vi "Begin.vi"(8 "error in":errorcluster) -> (0 "error out":errorcluster)   [LabVIEW 2020]
doc: "Called before other user functions, this VI is expected to open initial I/O refnums, load in file data, and do all program initialization. Notice that the <B>error out</B> terminal is simply used for data flow. Wiring it to other structures or subVIs ensures that this VI runs first."
uses:
  <vilib>/Rock Robotics/WPI/DriverStation/WPI_DriverStationRobotMode2.ctl
  <vilib>/Rock Robotics/WPI/Joystick/WPI_JoystickDeviceEnum.ctl
  <vilib>/Rock Robotics/WPI/ThirdParty/REV Robotics/REVLib/Typedef/Spark MAX Sensor Type.ctl
  <vilib>/Rock Robotics/WPI/SafetyOutput/WPI_SafetyOutputConfigMenu.ctl
  <vilib>/Rock Robotics/WPI/ThirdParty/REV Robotics/REVLib/Typedef/Spark MAX Motor Type.ctl
  Robot Global Data.vi
  <vilib>/Rock Robotics/Network Tables/NT Write String Array.vi
  <vilib>/Rock Robotics/WPI/RobotDrive/WPI_RobotDriveOpen2MotorWithExistingMotors.vi
  <vilib>/Rock Robotics/SystemInterfaces/DIO/FPGA_DIOPWMChannel.ctl
  <vilib>/Rock Robotics/WPI/RobotDrive/WPI_RobotDriveOpen2MotorWithVictorSPX.vi
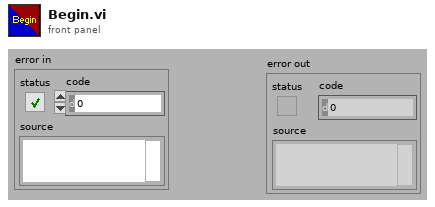
[diagram p1: front panel]
types:
  T1 = typedef "WPI_JoystickDeviceEnum.ctl" = enum16{"USB 0", "USB 1", "USB 2", "USB 3", "USB 4", "USB 5"}
  T2 = typedef "Spark MAX Motor Type.ctl" = enum16{"Brushed", "Brushless"}
  T3 = typedef "WPI_SafetyOutputConfigMenu.ctl" = enum16{"Enable", "Disable"}
  T4 = typedef "Spark MAX Sensor Type.ctl" = enum16{"No Sensor", "Hall Sensor", "Encoder", "-Not Available-", "Analog", "Alternate Encoder", "Duty Cycle"}
  T5 = typedef "WPI_DriverStationRobotMode2.ctl" = enum16{"Autonomous Disabled", "Autonomous Enabled", "Teleop Disabled", "Teleop Enabled", "Disconnected", "Finish", "Test Disabled", "Test Enabled", "Emergency Stopped"}
  T6 = typedef "FPGA_DIOPWMChannel.ctl" = enum8{"PWM 0", "PWM 1", "PWM 2", "PWM 3", "PWM 4", "PWM 5", "PWM 6", "PWM 7", "PWM 8", "PWM 9", "PWM MXP 0", "PWM MXP 1", "PWM MXP 2", "PWM MXP 3", "PWM MXP 4", "PWM MXP 5", "PWM MXP 6", "PWM MXP 7", "PWM MXP 8", "PWM MXP 9", "Invalid"}
  T7 = typedef "WPI_RobotDriveDevRef.ctl" = cluster{"DevStatus":errorcluster, "Motors[]":T8[], "Square Inputs":bool, "Max Output":dbl}
  T8 = typedef "WPI_MotorControlDeviceRef.ctl" = cluster{"DeviceStatus":errorcluster, "Type":T9, "PWM":cluster{"PWM Channel":T6, "DeadBand":T10}, "CAN":cluster{"Device Number":u8, "SetOutput VI Ref":variant, "GetOutput VI Ref":variant, "Enable VI Ref":variant, "Disable VI Ref":variant, "Data":variant}, "Invert":bool, "DIO PWM":cluster{"PWM \"Enable\" Channel":T6, "DIOChannel":T11, "PWM Rate":dbl}}
  T9 = typedef "WPI_MotorControlType.ctl" = enum16{"PWM", "CAN", "DIO PWM"}
  T10 = typedef "WPI_PWMDeadband.ctl" = cluster{"Name":string, "maxPositivePwm":i32, "minPositivePwm":i32, "centerPwm":i32, "maxNegativePwm":i32, "minNegativePwm":i32, "angularRange":u16}
  T11 = typedef "FPGA_DIOChannel.ctl" = enum8{"DIO 0", "DIO 1", "DIO 2", "DIO 3", "DIO 4", "DIO 5", "DIO 6", "DIO 7", "DIO 8", "DIO 9", "DIO MXP 0", "DIO MXP 1", "DIO MXP 2", "DIO MXP 3", "DIO MXP 4", "DIO MXP 5", "DIO MXP 6", "DIO MXP 7", "DIO MXP 8", "DIO MXP 9", "DIO MXP 10", "DIO MXP 11", "DIO MXP 12", "DIO MXP 13", "DIO MXP 14", "DIO MXP 15", "SPI Port CS1", "SPI Port CS2", "SPI Port CS3", "SPI Port MISO", "SPI Port MOSI", "Invalid"}
  T12 = typedef "WPI_JoystickDevRef.ctl" = cluster{"Device":T1}
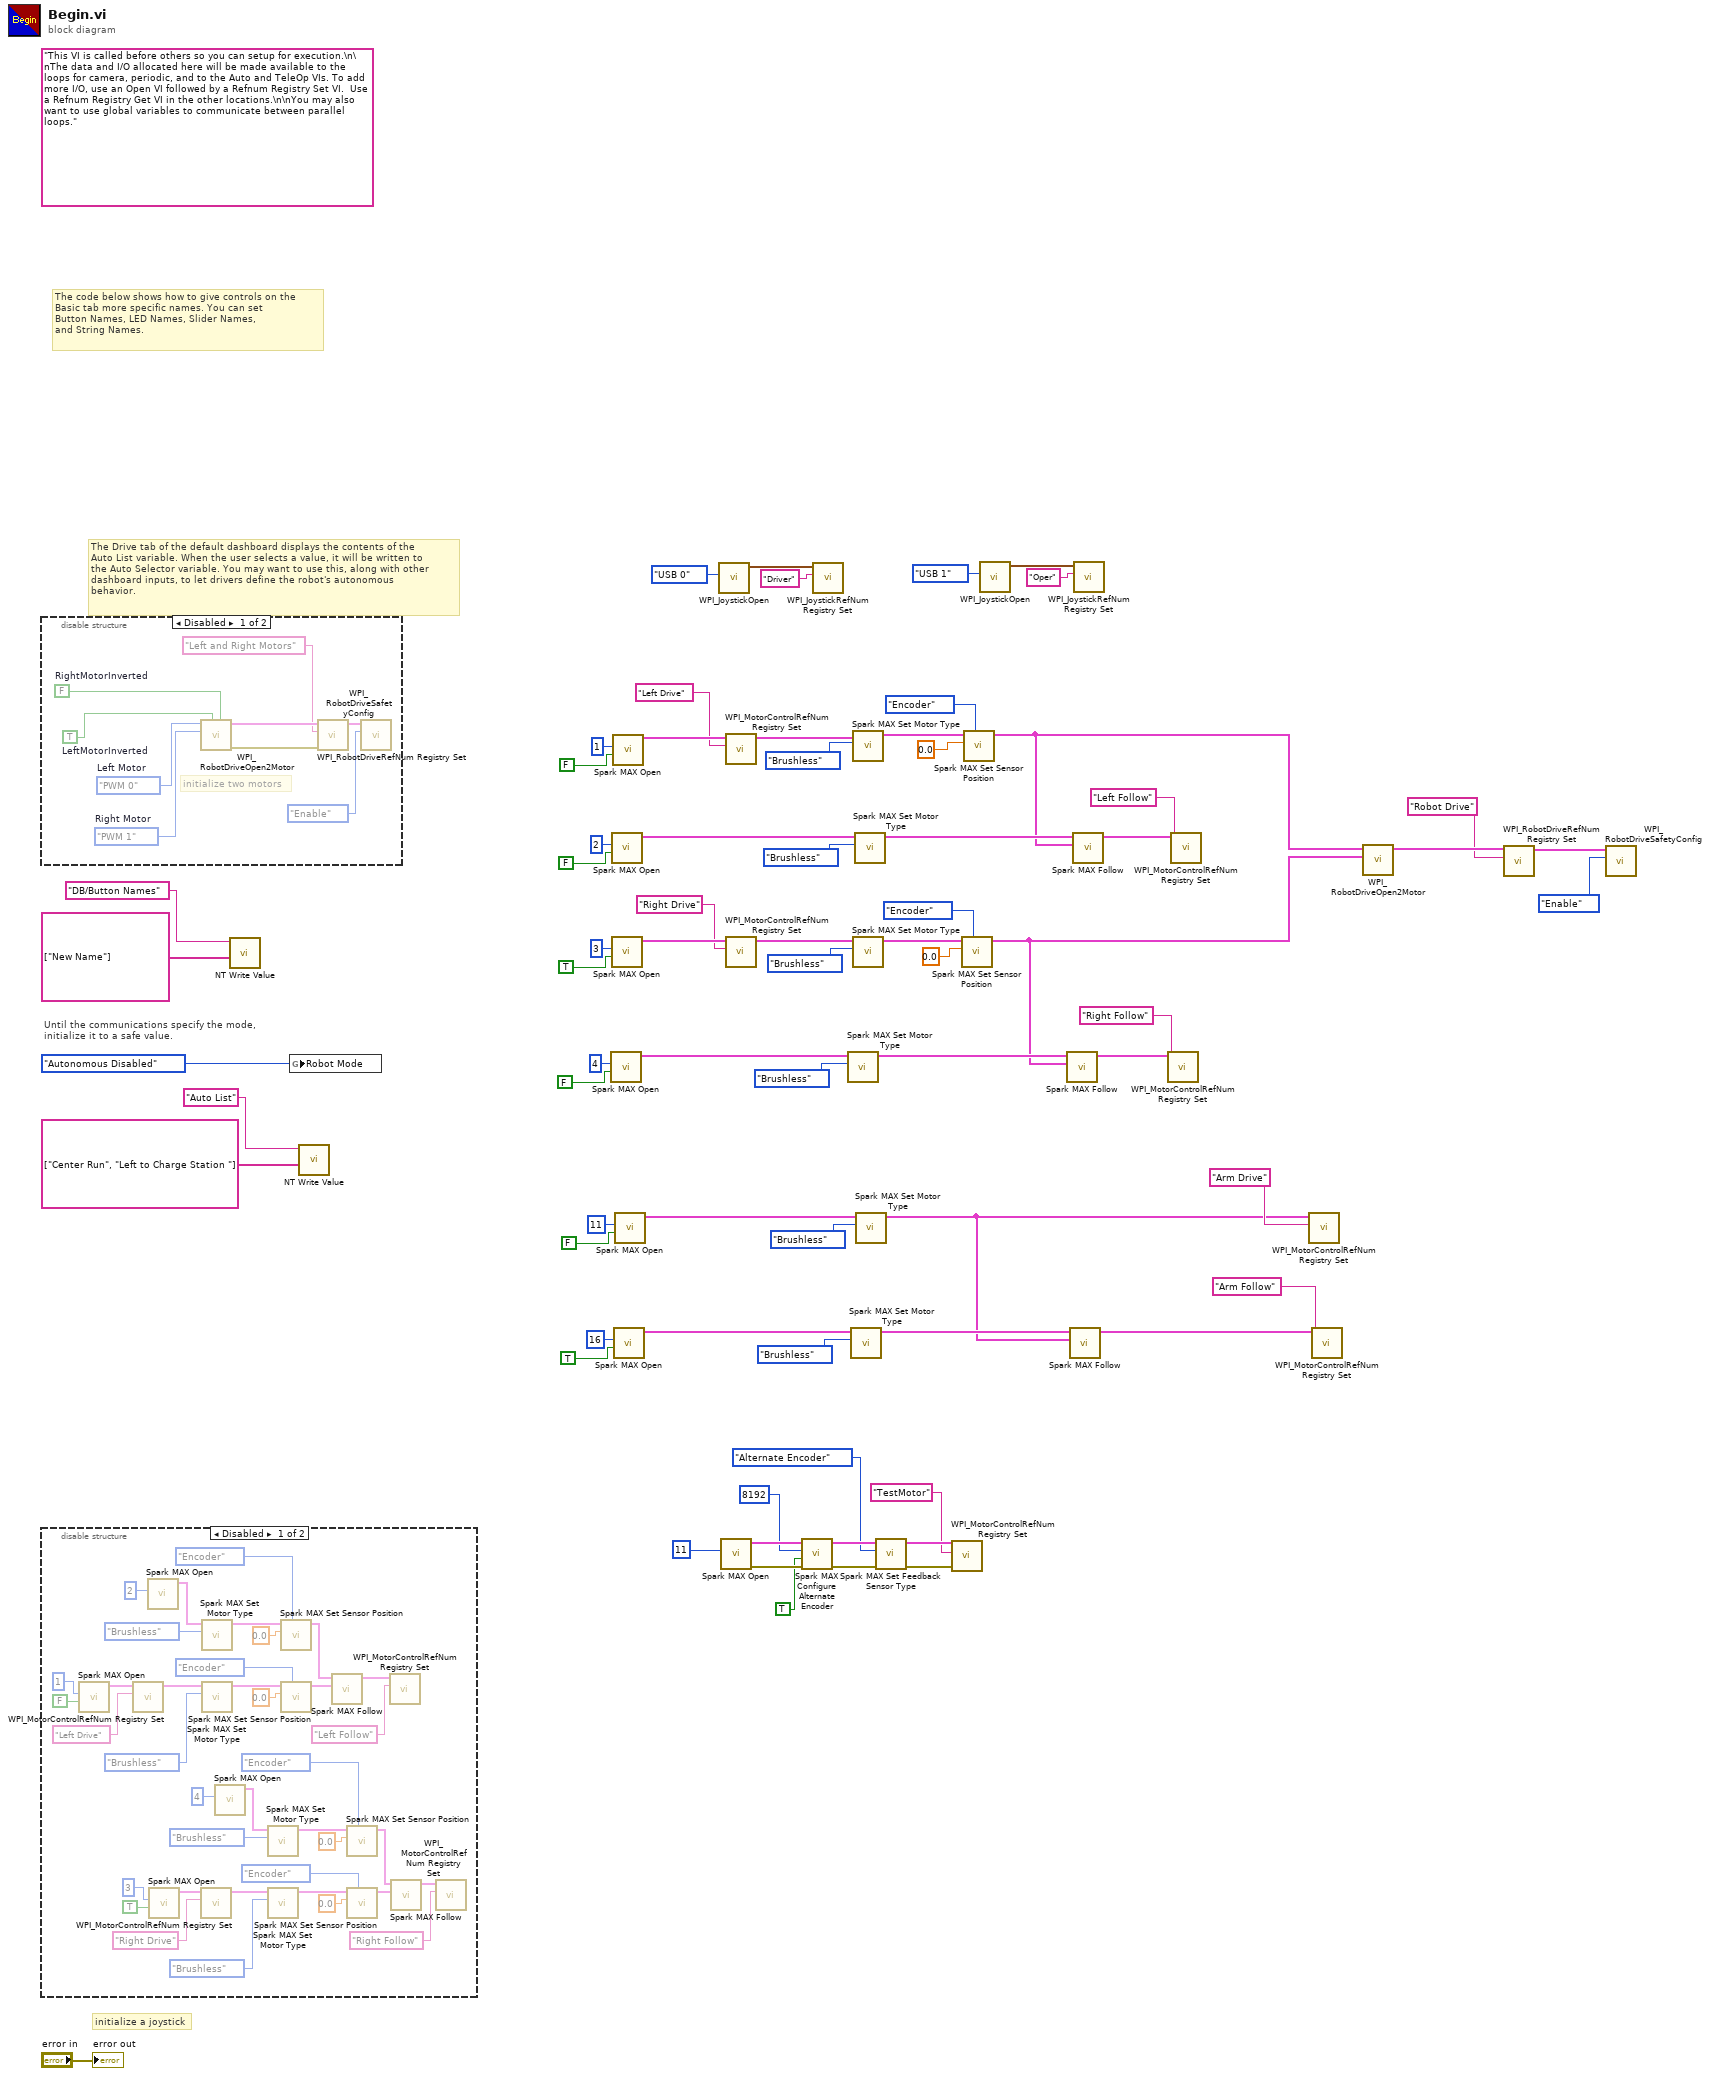
[diagram p0: block diagram]
diagram:
  (unwired) "This VI is called before others so you can setup for execution.\n\nThe data and I/O allocated here will be made available to the loops for camera, periodic, and to the Auto and TeleOp VIs. To add more I/O, use an Open VI followed by a Refnum Registry Set VI.  Use a Refnum Registry Get VI in the other locations.\n\nYou may also want to use global variables to communicate between parallel loops."
  # "initialize a joystick"
  # "The Drive tab of the default dashboard displays the contents of the\nAuto List variable. When the user selects a value, it will be written to\nthe Auto Selector variable. You may want to use this, along with other\ndashboard inputs, to let drivers define the robot's autonomous\nbehavior."
  # "The code below shows how to give controls on the\nBasic tab more specific names. You can set\nButton Names, LED Names, Slider Names,\nand String Names."
  # "Until the communications specify the mode,\ninitialize it to a safe value."
  n1 = disable-structure shown="Disabled" {
    frame Disabled {
      w77 = FPGA_DIOPWMChannel."PWM 1"  # Right Motor
      w78 = FPGA_DIOPWMChannel."PWM 0"  # Left Motor
      w82 = TRUE  # LeftMotorInverted
      w83 = FALSE  # RightMotorInverted
      # "initialize two motors"
      n2 = call-poly <vilib>:"WPI_RobotDriveOpen2Motor.vi"("Right Motor Inverted"=w83, "Left Motor Inverted"=w82, "Right Motor"=w77, "Left Motor"=w78) -> ("error out"=w79:errorcluster, "RobotDriveDevRef"=w81:T7)  [unwired: 1 in, 5 out]
      n3 = call <vilib>:"WPI_RobotDriveRefNum Registry Set.vi"("error in (no error)"=w79, "refnum name"="Left and Right Motors", "RobotDriveDevRef"=w81) -> ("RobotDriveDevRef"=w76:T7)  [unwired: 1 in, 7 out]
      n4 = call <vilib>:"WPI_RobotDriveSafetyConfig.vi"("mode"=WPI_SafetyOutputConfigMenu."Enable", "RobotDriveDevRef"=w76) -> ()  [unwired: 8 in, 2 out]
    }
    frame Enabled {
    }
  }
  n5 = disable-structure shown="Disabled" {
    frame Disabled {
      n6 = call <vilib>:"Spark MAX Open.vi"("Invert"=FALSE, "Device Number"=u8 1) -> ("MotorControlDeviceRef"=w116:T8)  [unwired: 8 in, 1 out]
      n7 = call <vilib>:"WPI_MotorControlRefNum Registry Set.vi"("refnum name"="Left Drive", "MotorControlDevRef"=w116) -> ("MotorControlDevRef"=w111:T8)  [unwired: 8 in, 1 out]
      n8 = call <vilib>:"Spark MAX Open.vi"("Device Number"=u8 2) -> ("MotorControlDeviceRef"=w108:T8)  [unwired: 9 in, 1 out]
      n9 = call <vilib>:"Spark MAX Open.vi"("Invert"=TRUE, "Device Number"=u8 3) -> ("MotorControlDeviceRef"=w114:T8)  [unwired: 8 in, 1 out]
      n10 = call <vilib>:"WPI_MotorControlRefNum Registry Set.vi"("refnum name"="Right Drive", "MotorControlDevRef"=w114) -> ("MotorControlDevRef"=w107:T8)  [unwired: 8 in, 1 out]
      n11 = call <vilib>:"Spark MAX Set Motor Type.vi"("Motor Type"=Spark_MAX_Motor_Type."Brushless", "MotorControlDevRef"=w108) -> ("MotorControlDeviceRef"=w97:T8)  [unwired: 8 in, 1 out]
      n12 = call <vilib>:"Spark MAX Set Motor Type.vi"("Motor Type"=Spark_MAX_Motor_Type."Brushless", "MotorControlDevRef"=w111) -> ("MotorControlDeviceRef"=w99:T8)  [unwired: 8 in, 1 out]
      n13 = call <vilib>:"Spark MAX Open.vi"("Device Number"=u8 4) -> ("MotorControlDeviceRef"=w105:T8)  [unwired: 9 in, 1 out]
      n14 = call <vilib>:"Spark MAX Set Motor Type.vi"("Motor Type"=Spark_MAX_Motor_Type."Brushless", "MotorControlDevRef"=w105) -> ("MotorControlDeviceRef"=w93:T8)  [unwired: 8 in, 1 out]
      n15 = call <vilib>:"Spark MAX Set Motor Type.vi"("Motor Type"=Spark_MAX_Motor_Type."Brushless", "MotorControlDevRef"=w107) -> ("MotorControlDeviceRef"=w95:T8)  [unwired: 8 in, 1 out]
      n16 = call <vilib>:"Spark MAX Set Sensor Position.vi"("Sensor Type (Hall Sensor)"=Spark_MAX_Sensor_Type."Encoder", "Position"=0.0, "MotorControlDeviceRef"=w97) -> ("MotorControlDeviceRef"=w91:T8)  [unwired: 7 in, 1 out]
      n17 = call <vilib>:"Spark MAX Set Sensor Position.vi"("Sensor Type (Hall Sensor)"=Spark_MAX_Sensor_Type."Encoder", "Position"=0.0, "MotorControlDeviceRef"=w99) -> ("MotorControlDeviceRef"=w88:T8)  [unwired: 7 in, 1 out]
      n18 = call <vilib>:"Spark MAX Follow.vi"("Master Controller"=w88, "MotorControlDeviceRef"=w91) -> ("MotorControlDeviceRef"=w87:T8)  [unwired: 8 in, 1 out]
      n19 = call <vilib>:"Spark MAX Set Sensor Position.vi"("Sensor Type (Hall Sensor)"=Spark_MAX_Sensor_Type."Encoder", "Position"=0.0, "MotorControlDeviceRef"=w93) -> ("MotorControlDeviceRef"=w90:T8)  [unwired: 7 in, 1 out]
      n20 = call <vilib>:"Spark MAX Set Sensor Position.vi"("Sensor Type (Hall Sensor)"=Spark_MAX_Sensor_Type."Encoder", "Position"=0.0, "MotorControlDeviceRef"=w95) -> ("MotorControlDeviceRef"=w89:T8)  [unwired: 7 in, 1 out]
      n21 = call <vilib>:"WPI_MotorControlRefNum Registry Set.vi"("refnum name"="Left Follow", "MotorControlDevRef"=w87) -> ()  [unwired: 8 in, 2 out]
      n22 = call <vilib>:"Spark MAX Follow.vi"("Master Controller"=w89, "MotorControlDeviceRef"=w90) -> ("MotorControlDeviceRef"=w86:T8)  [unwired: 8 in, 1 out]
      n23 = call <vilib>:"WPI_MotorControlRefNum Registry Set.vi"("refnum name"="Right Follow", "MotorControlDevRef"=w86) -> ()  [unwired: 8 in, 2 out]
    }
    frame Enabled {
    }
  }
  n24 = call-poly <vilib>:"NT Write Value.vi"("value"=string[] ["New Name"], "name"="DB/Button Names" ("Name")) -> ()  [unwired: 9 in, 1 out]
  n25 = global write "Robot Global Data.vi" "Robot Mode"(WPI_DriverStationRobotMode2."Autonomous Disabled" ("Robot Mode")) -> ()
  n26 = call-poly <vilib>:"NT Write Value.vi"("value"=string[] ["Center Run", "Left to Charge Station "] ("String Array"), "name"="Auto List" ("Name")) -> ()  [unwired: 9 in, 1 out]
  n27 = call <vilib>:"Spark MAX Open.vi"("Invert"=FALSE, "Device Number"=u8 4) -> ("MotorControlDeviceRef"=w37:T8)  [unwired: 8 in, 1 out]
  n28 = call <vilib>:"Spark MAX Open.vi"("Invert"=FALSE, "Device Number"=u8 2) -> ("MotorControlDeviceRef"=w41:T8)  [unwired: 8 in, 1 out]
  n29 = call <vilib>:"Spark MAX Open.vi"("Invert"=TRUE, "Device Number"=u8 3) -> ("MotorControlDeviceRef"=w47:T8)  [unwired: 8 in, 1 out]
  n30 = call <vilib>:"Spark MAX Open.vi"("Invert"=FALSE, "Device Number"=u8 1) -> ("MotorControlDeviceRef"=w46:T8)  [unwired: 8 in, 1 out]
  n31 = call <vilib>:"Spark MAX Open.vi"("Invert"=TRUE, "Device Number"=u8 16) -> ("MotorControlDeviceRef"=w12:T8)  [unwired: 8 in, 1 out]
  n32 = call <vilib>:"Spark MAX Open.vi"("Invert"=FALSE, "Device Number"=u8 11) -> ("MotorControlDeviceRef"=w7:T8)  [unwired: 8 in, 1 out]
  n33 = call <vilib>:"WPI_JoystickOpen.vi"("JoystickDevice"=WPI_JoystickDeviceEnum."USB 0") -> ("JoystickDevRef"=w68:T12)  [unwired: 10 in]
  n34 = call <vilib>:"Spark MAX Open.vi"("Device Number"=u8 11) -> ("error out"=w63:errorcluster, "MotorControlDeviceRef"=w64:T8)  [unwired: 9 in]
  n35 = call <vilib>:"WPI_MotorControlRefNum Registry Set.vi"("refnum name"="Left Drive", "MotorControlDevRef"=w46) -> ("MotorControlDevRef"=w43:T8)  [unwired: 8 in, 1 out]
  n36 = call <vilib>:"WPI_MotorControlRefNum Registry Set.vi"("refnum name"="Right Drive", "MotorControlDevRef"=w47) -> ("MotorControlDevRef"=w39:T8)  [unwired: 8 in, 1 out]
  n37 = call <vilib>:"Spark MAX Configure Alternate Encoder.vi"("error in (no error)"=w63, "Inverted (F)"=TRUE, "Cycles per Revolution (4096)"=u32 8192, "MotorControlDeviceRef in"=w64) -> ("error out"=w60:errorcluster, "MotorControlDeviceRef"=w61:T8)  [unwired: 6 in]
  n38 = call <vilib>:"WPI_JoystickRefNum Registry Set.vi"("refnum name"="Driver", "JoystickDevRef"=w68) -> ()  [unwired: 8 in, 2 out]
  n39 = call <vilib>:"Spark MAX Set Motor Type.vi"("Motor Type"=Spark_MAX_Motor_Type."Brushless", "MotorControlDevRef"=w37) -> ("MotorControlDeviceRef"=w28:T8)  [unwired: 8 in, 1 out]
  n40 = call <vilib>:"Spark MAX Set Motor Type.vi"("Motor Type"=Spark_MAX_Motor_Type."Brushless", "MotorControlDevRef"=w12) -> ("MotorControlDeviceRef"=w10:T8)  [unwired: 8 in, 1 out]
  n41 = call <vilib>:"Spark MAX Set Motor Type.vi"("Motor Type"=Spark_MAX_Motor_Type."Brushless", "MotorControlDevRef"=w43) -> ("MotorControlDeviceRef"=w35:T8)  [unwired: 8 in, 1 out]
  n42 = call <vilib>:"Spark MAX Set Motor Type.vi"("Motor Type"=Spark_MAX_Motor_Type."Brushless", "MotorControlDevRef"=w39) -> ("MotorControlDeviceRef"=w32:T8)  [unwired: 8 in, 1 out]
  n43 = call <vilib>:"Spark MAX Set Motor Type.vi"("Motor Type"=Spark_MAX_Motor_Type."Brushless", "MotorControlDevRef"=w41) -> ("MotorControlDeviceRef"=w29:T8)  [unwired: 8 in, 1 out]
  n44 = call <vilib>:"Spark MAX Set Motor Type.vi"("Motor Type"=Spark_MAX_Motor_Type."Brushless", "MotorControlDevRef"=w7) -> ("MotorControlDeviceRef"=w5:T8)  [unwired: 8 in, 1 out]
  n45 = call <vilib>:"Spark MAX Set Feedback Sensor Type.vi"("error in (no error)"=w60, "Sensor Type"=Spark_MAX_Sensor_Type."Alternate Encoder", "MotorControlDevRef"=w61) -> ("error out"=w57:errorcluster, "MotorControlDeviceRef"=w58:T8)  [unwired: 7 in]
  n46 = call <vilib>:"WPI_MotorControlRefNum Registry Set.vi"("error in (no error)"=w57, "refnum name"="TestMotor", "MotorControlDevRef"=w58) -> ()  [unwired: 7 in, 2 out]
  n47 = call <vilib>:"Spark MAX Set Sensor Position.vi"("Sensor Type (Hall Sensor)"=Spark_MAX_Sensor_Type."Encoder", "Position"=0.0, "MotorControlDeviceRef"=w32) -> ("MotorControlDeviceRef"=w22:T8)  [unwired: 7 in, 1 out]
  n48 = call <vilib>:"Spark MAX Set Sensor Position.vi"("Sensor Type (Hall Sensor)"=Spark_MAX_Sensor_Type."Encoder", "Position"=0.0, "MotorControlDeviceRef"=w35) -> ("MotorControlDeviceRef"=w23:T8)  [unwired: 7 in, 1 out]
  n49 = call <vilib>:"WPI_JoystickOpen.vi"("JoystickDevice"=WPI_JoystickDeviceEnum."USB 1") -> ("JoystickDevRef"=w2:T12)  [unwired: 10 in]
  n50 = call <vilib>:"Spark MAX Follow.vi"("Master Controller"=w22, "MotorControlDeviceRef"=w28) -> ("MotorControlDeviceRef"=w25:T8)  [unwired: 8 in, 1 out]
  n51 = call <vilib>:"Spark MAX Follow.vi"("Master Controller"=w5, "MotorControlDeviceRef"=w10) -> ("MotorControlDeviceRef"=w9:T8)  [unwired: 8 in, 1 out]
  n52 = call <vilib>:"Spark MAX Follow.vi"("Master Controller"=w23, "MotorControlDeviceRef"=w29) -> ("MotorControlDeviceRef"=w27:T8)  [unwired: 8 in, 1 out]
  n53 = call <vilib>:"WPI_JoystickRefNum Registry Set.vi"("refnum name"="Oper", "JoystickDevRef"=w2) -> ()  [unwired: 8 in, 2 out]
  n54 = call <vilib>:"WPI_MotorControlRefNum Registry Set.vi"("refnum name"="Right Follow", "MotorControlDevRef"=w25) -> ()  [unwired: 8 in, 2 out]
  n55 = call <vilib>:"WPI_MotorControlRefNum Registry Set.vi"("refnum name"="Left Follow", "MotorControlDevRef"=w27) -> ()  [unwired: 8 in, 2 out]
  n56 = call <vilib>:"WPI_MotorControlRefNum Registry Set.vi"("refnum name"="Arm Drive", "MotorControlDevRef"=w5) -> ()  [unwired: 8 in, 2 out]
  n57 = call <vilib>:"WPI_MotorControlRefNum Registry Set.vi"("refnum name"="Arm Follow", "MotorControlDevRef"=w9) -> ()  [unwired: 8 in, 2 out]
  n58 = call-poly <vilib>:"WPI_RobotDriveOpen2Motor.vi"("Right Motor Dev Ref"=w22, "Left Motor Dev Ref"=w23) -> ("RobotDriveDevRef"=w21:T7)  [unwired: 3 in, 6 out]
  n59 = call <vilib>:"WPI_RobotDriveRefNum Registry Set.vi"("refnum name"="Robot Drive", "RobotDriveDevRef"=w21) -> ("RobotDriveDevRef"=w19:T7)  [unwired: 8 in, 1 out]
  n60 = call <vilib>:"WPI_RobotDriveSafetyConfig.vi"("mode"=WPI_SafetyOutputConfigMenu."Enable", "RobotDriveDevRef"=w19) -> ()  [unwired: 8 in, 2 out]
  "error out" <- "error in"
